vi "MUX80_Split_Page_Range.vi"(0 "Array In":u16[](array[ring]) items=["LJ_rgBIP10V", "LJ_rgBIP5V", "LJ_rgUNI5V", "LJ_rgUNI2P5V", "LJ_rgUNI1P25V", "LJ_rgBIP1V", "LJ_rgUNIP625V", "LJ_rgBIPP1V", "LJ_rgBIPP01V"]) -> (1 "Page 1 out":u16[](array[ring]) items=["LJ_rgBIP10V", "LJ_rgBIP5V", "LJ_rgUNI5V", "LJ_rgUNI2P5V", "LJ_rgUNI1P25V", "LJ_rgBIP1V", "LJ_rgUNIP625V", "LJ_rgBIPP1V", "LJ_rgBIPP01V"], 2 "Page 6 out":u16[](array[ring]) items=["LJ_rgBIP10V", "LJ_rgBIP5V", "LJ_rgUNI5V", "LJ_rgUNI2P5V", "LJ_rgUNI1P25V", "LJ_rgBIP1V", "LJ_rgUNIP625V", "LJ_rgBIPP1V", "LJ_rgBIPP01V"], 3 "Page 2 out":u16[](array[ring]) items=["LJ_rgBIP10V", "LJ_rgBIP5V", "LJ_rgUNI5V", "LJ_rgUNI2P5V", "LJ_rgUNI1P25V", "LJ_rgBIP1V", "LJ_rgUNIP625V", "LJ_rgBIPP1V", "LJ_rgBIPP01V"], 4 "Page 3 out":u16[](array[ring]) items=["LJ_rgBIP10V", "LJ_rgBIP5V", "LJ_rgUNI5V", "LJ_rgUNI2P5V", "LJ_rgUNI1P25V", "LJ_rgBIP1V", "LJ_rgUNIP625V", "LJ_rgBIPP1V", "LJ_rgBIPP01V"], 5 "Page 4 out":u16[](array[ring]) items=["LJ_rgBIP10V", "LJ_rgBIP5V", "LJ_rgUNI5V", "LJ_rgUNI2P5V", "LJ_rgUNI1P25V", "LJ_rgBIP1V", "LJ_rgUNIP625V", "LJ_rgBIPP1V", "LJ_rgBIPP01V"], 6 "Page 5 out":u16[](array[ring]) items=["LJ_rgBIP10V", "LJ_rgBIP5V", "LJ_rgUNI5V", "LJ_rgUNI2P5V", "LJ_rgUNI1P25V", "LJ_rgBIP1V", "LJ_rgUNIP625V", "LJ_rgBIPP1V", "LJ_rgBIPP01V"])   [LabVIEW 2020]
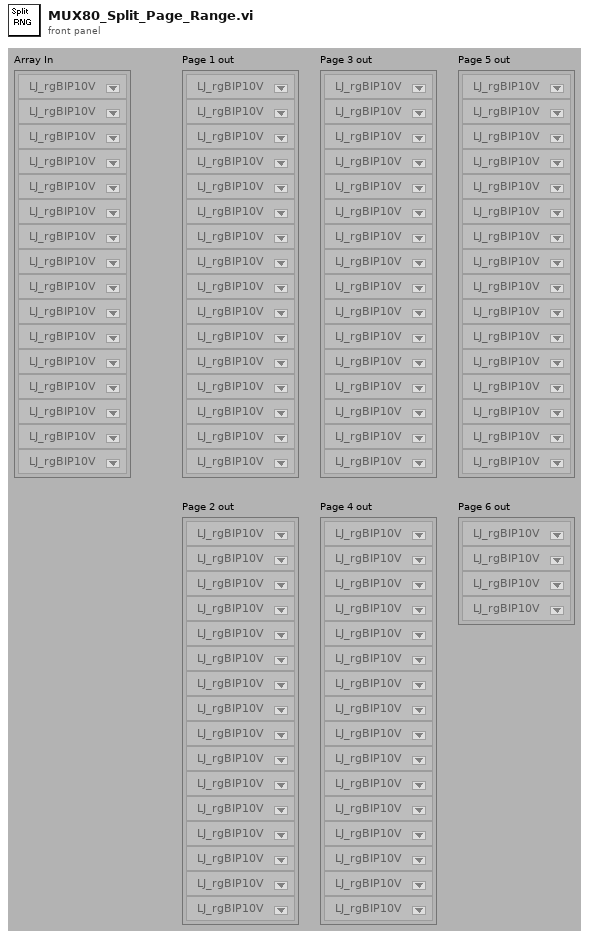
[diagram p1: front panel]
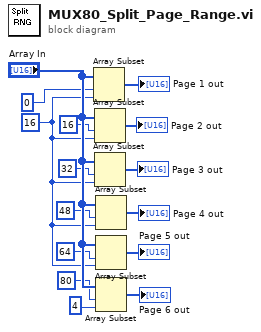
[diagram p0: block diagram]
diagram:
  w7 = 16
  n1 = Array Subset(array="Array In", index=0, length=w7) -> (→"Page 1 out":u16[])
  n2 = Array Subset(array="Array In", index=16, length=w7) -> (→"Page 2 out":u16[])
  n3 = Array Subset(array="Array In", index=32, length=w7) -> (→"Page 3 out":u16[])
  n4 = Array Subset(array="Array In", index=48, length=w7) -> (→"Page 4 out":u16[])
  n5 = Array Subset(array="Array In", index=64, length=w7) -> (→"Page 5 out":u16[])
  n6 = Array Subset(array="Array In", index=80, length=4) -> (→"Page 6 out":u16[])
